vi "Resize Window.vi"(8 "error in (no error)":errorcluster, 10 "Focus":enum8{"FP", "BD"}(ring), 11 "VI Refnum in":refnum<vi>) -> (0 "error out":errorcluster, 3 "VI Refnum out":refnum<vi>)   [LabVIEW 2019, in "Builtins.lvlib"]
doc: "Resizes the front panel or block diagram window to content. On the front panel, this also resets the origins to 0, 0.\n\nCreated by: Ryan Pacini"
uses:
  Builtins.lvlib
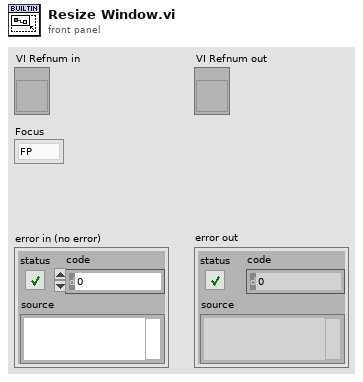
[diagram p1: front panel]
types:
  T1 = typedef "LVAllMonitorsDisplayTypeDef.ctl" = cluster{"Bounds":cluster{"Left":i16, "Top":i16, "Right":i16, "Bottom":i16}, "Depth":i16}[]
  T2 = cluster{"Left":i16, "Top":i16, "Right":i16, "Bottom":i16}
  T3 = typedef "LVRectTypeDef.ctl" = cluster{"Left":i16, "Top":i16, "Right":i16, "Bottom":i16}
  T4 = typedef "LVBoundsTypeDef.ctl" = cluster{"Width":u32, "Height":u32}
  T5 = typedef "LVPointTypeDef.ctl" = cluster{"Horizontal":i16, "Vertical":i16}
  T6 = typedef "LVPositionTypeDef.ctl" = cluster{"Left":i32, "Top":i32}
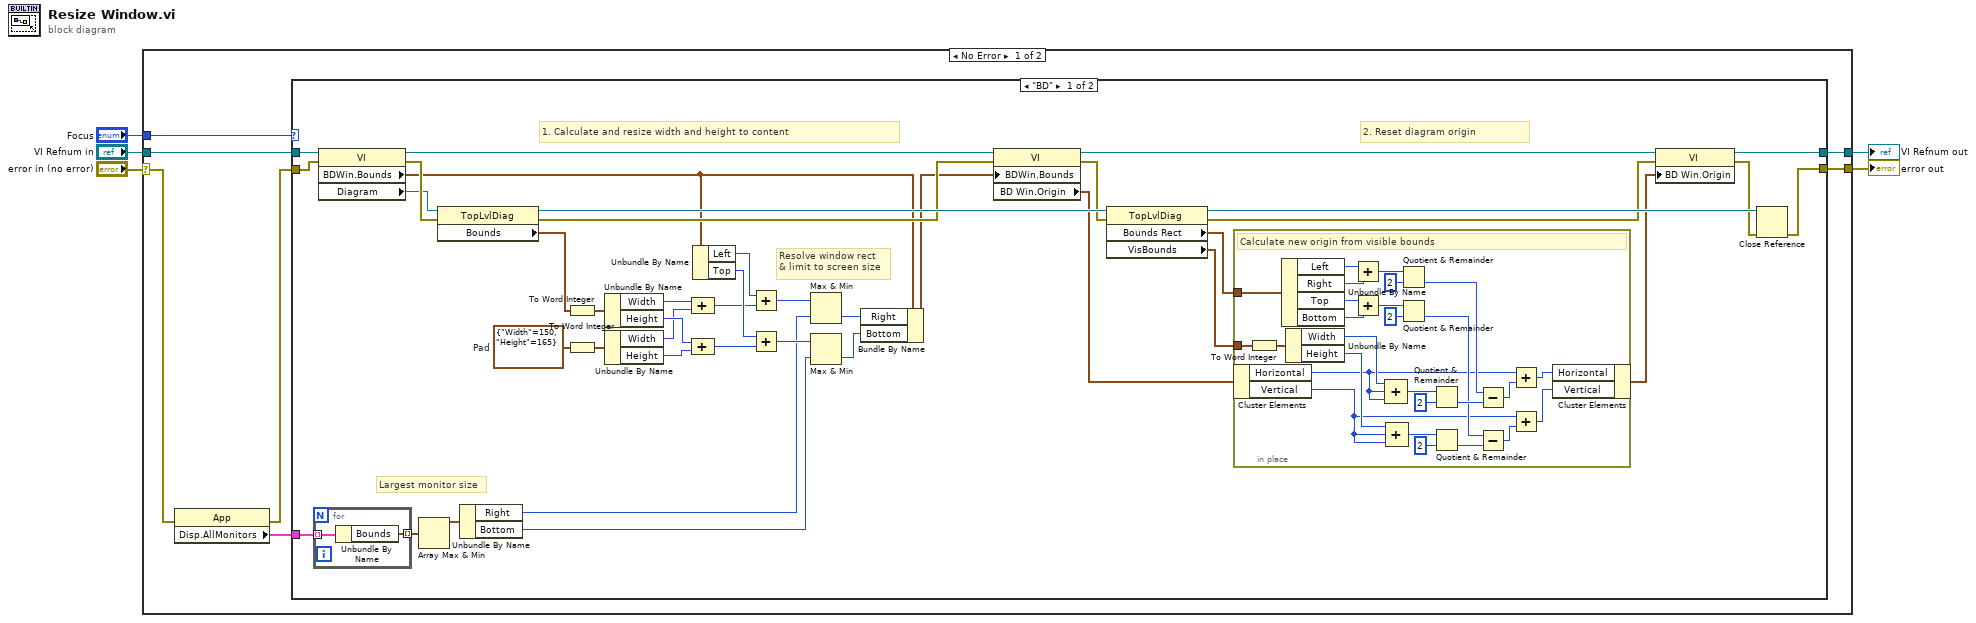
[diagram p0: block diagram]
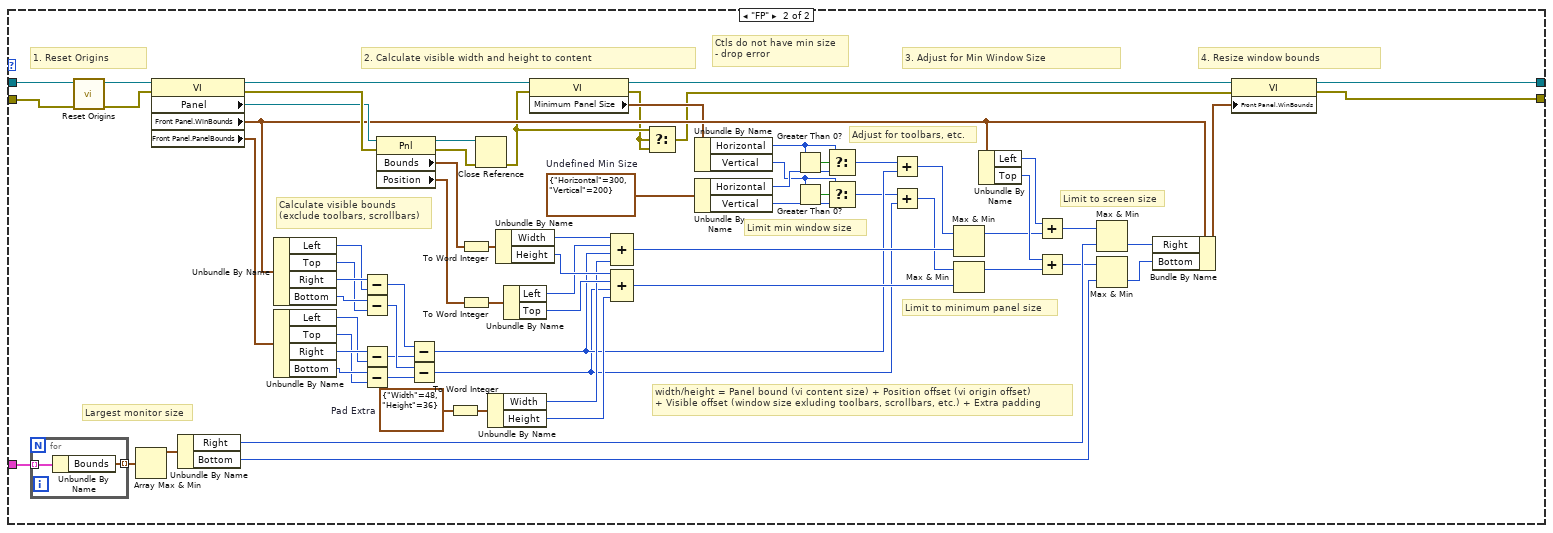
[diagram p2: hidden frame]
diagram:
  n1 = case shown="No Error" "error in (no error)" {
    selector: "error in (no error)" -> [w7 w156]
    tunnel: [w12 w157] -> w5
    tunnel: "VI Refnum in" -> [w11 w157]
    tunnel: [w10 w156] -> w2
    tunnel: "Focus" -> [w9 _]
    frame No Error {
      n2 = property class="App"(error in=w7) -> (error out=w6:errorcluster, "Disp.AllMonitors"=w8:T1)  [unwired: 1 in, 1 out]
      n3 = case shown="\"BD\"" w9 {
        tunnel: [w53 w153] -> w12
        tunnel: w11 -> [w52 w110]
        tunnel: w6 -> [w51 w112]
        tunnel: [w36 w108] -> w10
        tunnel: w8 -> [w14 w114]
        frame "BD" {
          w17 = cluster{"Width":u32, "Height":u32} {"Width"=150, "Height"=165}  # Pad
          # "Largest monitor size"
          # "2. Reset diagram origin"
          # "1. Calculate and resize width and height to content"
          # "Resolve window rect\n& limit to screen size"
          n4 = for {
            tunnel: w14 -> [w82] mode=indexing
            tunnel: [w81] -> w37 mode=indexing
            n5 = Unbundle By Name(w82) -> ("Bounds"=w81:T2)
          }
          n6 = property on="Property Node" class="VI"(reference=w52, error in=w51) -> (reference out=w13:refnum<vi>, error out=w43:errorcluster, "BDWin.Bounds"=w25:T3, "Diagram"=w19:refnum<vi>)
          n7 = Array Max & Min(array=w37) -> (max value=w44:T2)  [unwired: 3 out]
          n8 = property on="Property Node" class="TopLvlDiag"(reference=w19, error in=w43) -> (reference out=w49:refnum<vi>, error out=w42:errorcluster, "Bounds"=w34:T4)
          n9 = Unbundle By Name(w44) -> ("Right"=w22:i16, "Bottom"=w21:i16)
          n10 = To Word Integer(number=w34) -> (16bit integer=w35:cluster{"Width":i16, "Height":i16})
          n11 = To Word Integer(number=w17) -> (16bit integer=w18:cluster{"Width":i16, "Height":i16})
          n12 = Unbundle By Name(w35) -> ("Width"=w32:i16, "Height"=w33:i16)
          n13 = Unbundle By Name(w18) -> ("Width"=w15:i16, "Height"=w16:i16)
          n14 = Compound Arithmetic op=ADD(w32, w15) -> (w24:i16)
          n15 = Compound Arithmetic op=ADD(w33, w16) -> (w23:i16)
          n16 = Unbundle By Name(w25) -> ("Left"=w29:i16, "Top"=w26:i16)
          n17 = Add(x=w29, y=w24) -> (x+y=w28:i16)
          n18 = Add(x=w26, y=w23) -> (x+y=w27:i16)
          n19 = Max & Min(x=w28, y=w22) -> (min(x,y)=w30:i16)  [unwired: 1 out]
          n20 = Max & Min(x=w27, y=w21) -> (min(x,y)=w31:i16)  [unwired: 1 out]
          n21 = Bundle By Name(cluster=w25, "Right"=w30, "Bottom"=w31) -> (w20:T3)
          n22 = property on="Property Node" class="VI"(reference=w13, error in=w42, "BDWin.Bounds"=w20) -> (reference out=w48:refnum<vi>, error out=w41:errorcluster, "BD Win.Origin"=w46:T5)
          n23 = property on="Property Node" class="TopLvlDiag"(reference=w49, error in=w41) -> (reference out=w50:refnum<vi>, error out=w39:errorcluster, "Bounds Rect"=w40:T3, "VisBounds"=w45:T4)
          n24 = in-place {
            in-place-border: w40 -> [w76]
            in-place-border: w45 -> [w64]
            # "Calculate new origin from visible bounds"
            n25 = in-place-cluster #1(w46) -> ("Horizontal"=w58:i16, "Vertical"=w57:i16)
            n26 = To Word Integer(number=w64) -> (16bit integer=w63:cluster{"Width":i16, "Height":i16})
            n27 = Unbundle By Name(w76) -> ("Left"=w80:i16, "Right"=w79:i16, "Top"=w78:i16, "Bottom"=w77:i16)
            n28 = Unbundle By Name(w63) -> ("Width"=w60:i16, "Height"=w62:i16)
            n29 = Add(x=w80, y=w79) -> (x+y=w75:i16)
            n30 = Add(x=w78, y=w77) -> (x+y=w74:i16)
            n31 = Compound Arithmetic op=ADD(w60, w58, w58) -> (w59:i16)
            n32 = Compound Arithmetic op=ADD(w62, w57, w57) -> (w61:i16)
            n33 = Quotient & Remainder(x=w75, y=i16 2) -> (floor(x/y)=w70:i16)  [unwired: 1 out]
            n34 = Quotient & Remainder(x=w74, y=i16 2) -> (floor(x/y)=w67:i16)  [unwired: 1 out]
            n35 = Quotient & Remainder(x=w59, y=i16 2) -> (floor(x/y)=w71:i16)  [unwired: 1 out]
            n36 = Quotient & Remainder(x=w61, y=i16 2) -> (floor(x/y)=w69:i16)  [unwired: 1 out]
            n37 = Subtract(x=w70, y=w71) -> (x-y=w66:i16)
            n38 = Subtract(x=w67, y=w69) -> (x-y=w65:i16)
            n39 = Add(x=w58, y=w66) -> (x+y=w56:i16)
            n40 = Add(x=w57, y=w65) -> (x+y=w55:i16)
            n41 = in-place-cluster #1("Horizontal"=w56, "Vertical"=w55) -> (w47:T5)
          }
          n42 = property on="Property Node" class="VI"(reference=w48, error in=w39, "BD Win.Origin"=w47) -> (reference out=w53:refnum<vi>, error out=w38:errorcluster)
          n43 = Close Reference(reference=w50, error in (no error)=w38) -> (error out=w36:errorcluster)
        }
        frame "FP" {
          w94 = cluster{"Horizontal":i16, "Vertical":i16} {"Horizontal"=300, "Vertical"=200}  # Undefined Min Size
          w117 = cluster{"Width":u32, "Height":u32} {"Width"=48, "Height"=36}  # Pad Extra
          # "Ctls do not have min size\n- drop error"
          # "width/height = Panel bound (vi content size) + Position offset (vi origin offset)\n+ Visible offset (window size exluding toolbars, scrollbars, etc.) + Extra padding"
          # "4. Resize window bounds"
          # "3. Adjust for Min Window Size"
          # "Adjust for toolbars, etc."
          # "Limit min window size"
          # "Limit to minimum panel size"
          # "Largest monitor size"
          # "Calculate visible bounds\n(exclude toolbars, scrollbars)"
          # "1. Reset Origins"
          # "2. Calculate visible width and height to content"
          # "Limit to screen size"
          n44 = for {
            tunnel: w114 -> [w155] mode=indexing
            tunnel: [w154] -> w142 mode=indexing
            n45 = Unbundle By Name(w155) -> ("Bounds"=w154:T2)
          }
          n46 = call "Reset Origins.vi"("error in (no error)"=w112, "VI Refnum in"=w110) -> ("error out"=w113:errorcluster, "VI Refnum out"=w111:refnum<vi>)  [unwired: 8 in]
          n47 = Array Max & Min(array=w142) -> (max value=w151:T2)  [unwired: 3 out]
          n48 = property on="Property Node" class="VI"(reference=w111, error in=w113) -> (reference out=w105:refnum<vi>, error out=w148:errorcluster, "Panel"=w145:refnum<vi>, "Front Panel.WinBounds"=w131:T3, "Front Panel.PanelBounds"=w141:T3)
          n49 = Unbundle By Name(w151) -> ("Right"=w143:i16, "Bottom"=w144:i16)
          n50 = Unbundle By Name(w131) -> ("Left"=w126:i16, "Top"=w124:i16, "Right"=w128:i16, "Bottom"=w127:i16)
          n51 = Unbundle By Name(w141) -> ("Left"=w122:i16, "Top"=w120:i16, "Right"=w130:i16, "Bottom"=w129:i16)
          n52 = Subtract(x=w128, y=w126) -> (x-y=w125:i16)
          n53 = Subtract(x=w127, y=w124) -> (x-y=w123:i16)
          n54 = Subtract(x=w130, y=w122) -> (x-y=w121:i16)
          n55 = Subtract(x=w129, y=w120) -> (x-y=w119:i16)
          n56 = property on="Property Node" class="Pnl"(reference=w145, error in=w148) -> (reference out=w107:refnum<vi>, error out=w106:errorcluster, "Bounds"=w147:T4, "Position"=w109:T6)
          n57 = Subtract(x=w125, y=w121) -> (x-y=w98:i16)
          n58 = Subtract(x=w123, y=w119) -> (x-y=w95:i16)
          n59 = To Word Integer(number=w117) -> (16bit integer=w118:cluster{"Width":i16, "Height":i16})
          n60 = To Word Integer(number=w147) -> (16bit integer=w152:cluster{"Width":i16, "Height":i16})
          n61 = To Word Integer(number=w109) -> (16bit integer=w137:cluster{"Left":i16, "Top":i16})
          n62 = Close Reference(reference=w107, error in (no error)=w106) -> (error out=w85:errorcluster)
          n63 = Unbundle By Name(w118) -> ("Width"=w116:i16, "Height"=w115:i16)
          n64 = Unbundle By Name(w152) -> ("Width"=w140:i16, "Height"=w139:i16)
          n65 = Unbundle By Name(w137) -> ("Left"=w138:i16, "Top"=w136:i16)
          n66 = property class="VI"(reference=w105, error in=w85) -> (reference out=w104:refnum<vi>, error out=w84:errorcluster, "Minimum Panel Size"=w103:T5)
          n67 = Compound Arithmetic op=ADD(w140, w138, w98, w116) -> (w102:i16)
          n68 = Compound Arithmetic op=ADD(w139, w136, w95, w115) -> (w100:i16)
          n69 = Select(t=w85, s=w84, f=w84) -> (s? t:f=w83:errorcluster)
          n70 = Unbundle By Name(w103) -> ("Horizontal"=w92:i16, "Vertical"=w88:i16)
          n71 = Unbundle By Name(w94) -> ("Horizontal"=w90:i16, "Vertical"=w87:i16)
          n72 = Greater Than 0?(x=w92) -> (x > 0?=w93:bool)
          n73 = Greater Than 0?(x=w88) -> (x > 0?=w89:bool)
          n74 = Select(t=w92, s=w93, f=w90) -> (s? t:f=w91:i16)
          n75 = Select(t=w88, s=w89, f=w87) -> (s? t:f=w86:i16)
          n76 = Add(x=w91, y=w98) -> (x+y=w97:i16)
          n77 = Add(x=w86, y=w95) -> (x+y=w96:i16)
          n78 = Max & Min(x=w97, y=w102) -> (max(x,y)=w101:i16)  [unwired: 1 out]
          n79 = Max & Min(x=w96, y=w100) -> (max(x,y)=w99:i16)  [unwired: 1 out]
          n80 = Unbundle By Name(w131) -> ("Left"=w135:i16, "Top"=w132:i16)
          n81 = Add(x=w135, y=w101) -> (x+y=w134:i16)
          n82 = Add(x=w132, y=w99) -> (x+y=w133:i16)
          n83 = Max & Min(x=w134, y=w143) -> (min(x,y)=w149:i16)  [unwired: 1 out]
          n84 = Max & Min(x=w133, y=w144) -> (min(x,y)=w150:i16)  [unwired: 1 out]
          n85 = Bundle By Name(cluster=w131, "Right"=w149, "Bottom"=w150) -> (w146:T3)
          n86 = property on="Property Node" class="VI"(reference=w104, error in=w83, "Front Panel.WinBounds"=w146) -> (reference out=w153:refnum<vi>, error out=w108:errorcluster)
        }
      }
    }
    frame Error {
    }
  }
  "VI Refnum out" <- w5
  "error out" <- w2
